vi "Facade.vi"(0 "Data In":T10 {"Duration (s)" format="%<%M:%S>T"}, 2 "Display State In":T8, 3 "Container State":T9) -> (6 "Data Out":T10 {"Duration (s)" format="%<%M:%S>T"}, 7 "Display State Out":T8, 8 "Action":T7)   [LabVIEW 2015, in "Song Browser.lvlib" / "Song Browser.xctl"]
uses:
  Song Browser.xctl
  Data.ctl
  controls/Queue Song Display.ctl
  file/MusicElement/Song/Song Duration.ctl
  controls/Dequeue Control.ctl
  <vilib>/_xctls/Container State.ctl
  State.ctl
  controls/Song Browser Display.ctl
  controls/Enqueue Control.ctl
  <vilib>/_xctls/Action.ctl
  controls/Ascending_Descending Order.ctl
  file/MusicElement/MusicElementLibrary/SongLibrary/Song Display Sort Option.ctl
  <vilib>/_xctls/XControlSupport.lvlib
  file/MusicElement/MusicElementLibrary/SongLibrary/SongLibrary.lvclass
  file/MusicElement/Song/Song.lvclass
panel:
  in  "Remove Filters":bool
  in  "Time Sort":bool
  out "Sort Time Indicator":T1
  out "Sort Album Indicator":T1
  in  "Album Sort":bool
  out "Sort Artist Indicator":T1
  in  "Artist Sort":bool
  in  "Song Sort":bool
  out "Sort Songs Indicator":T1
  out "Unfiltered Array":T2[](array[typedef]) {"Duration (s)" format="%<%M:%S>T"}
  in  "Array":T5[](array[typedef]) {"Duration (s)" format="%<%M:%S>T"}
  in  "Scrollbar":i32(c297)
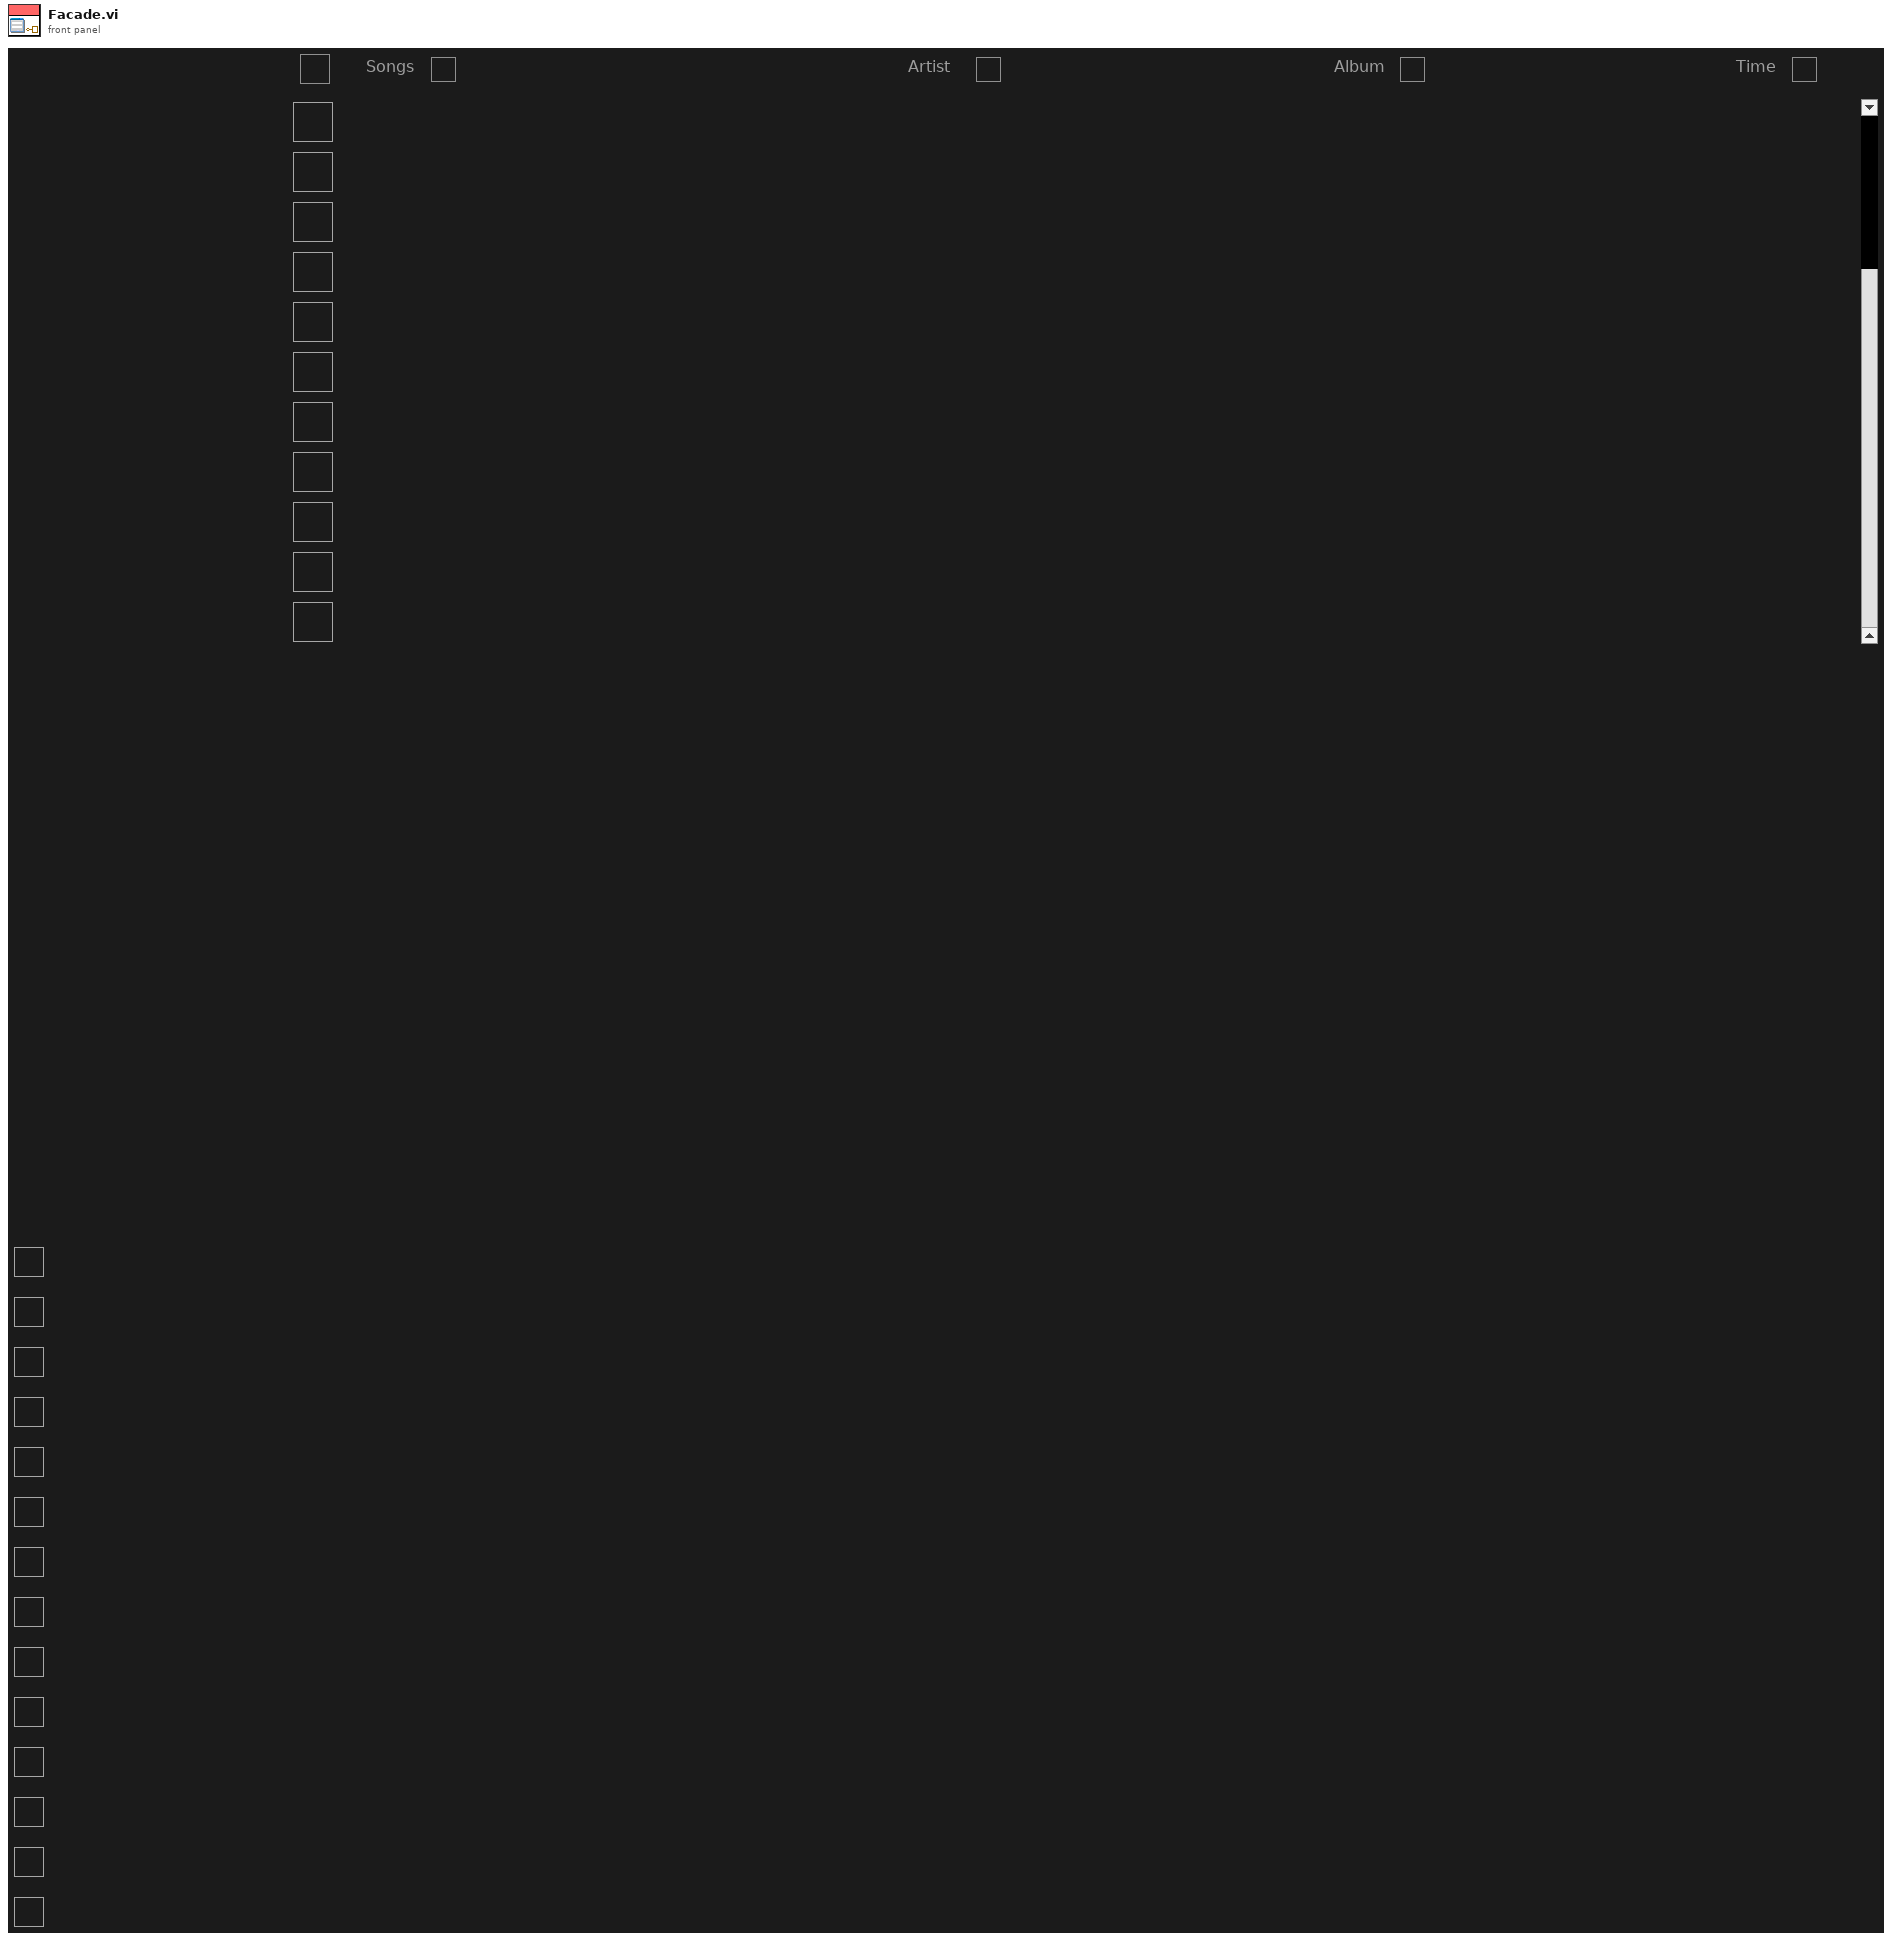
[diagram p1: front panel]
types:
  T1 = typedef "Ascending_Descending Order.ctl" = bool
  T2 = typedef "Queue Song Display.ctl" = cluster{"Song Name":string, "Artist":string, "Album":string, "Duration (s)":T3, "UID":string, "Dequeue":T4}
  T3 = typedef "Song.lvclass/Song Duration.ctl" = timestamp
  T4 = typedef "Dequeue Control.ctl" = bool
  T5 = typedef "Song Browser Display.ctl" = cluster{"Song Name":string, "Artist":string, "Album":string, "Duration (s)":T3, "UID":string, "Enqueue":T6}
  T6 = typedef "Enqueue Control.ctl" = bool
  T7 = typedef "XControlSupport.lvlib/Action.ctl" = cluster{"Data Changed?":bool, "State Changed?":bool, "Action Name":string}
  T8 = typedef "Song Browser.lvlib/Song Browser.xctl/State.ctl" = cluster{"Element Selected Event":refnum<user-event>}
  T9 = typedef "XControlSupport.lvlib/Container State.ctl" = cluster{"Indicator?":bool, "Run Mode?":bool, " Refnum":refnum<vi>}
  T10 = typedef "Song Browser.lvlib/Song Browser.xctl/Data.ctl" = T2[]
  T11 = cluster{"Song Name":bool, "Artist":bool, "Album":bool, "Duration (s)":bool, "UID":bool, "Enqueue":T6}
  T12 = typedef "SongLibrary.lvclass/Song Display Sort Option.ctl" = enum16{"Song", "Artist", "Album", "Time"}
  T13 = cluster{"Song Name":bool, "Artist":bool, "Album":bool, "Duration (s)":bool, "UID":bool, "Enqueue":T6}[]
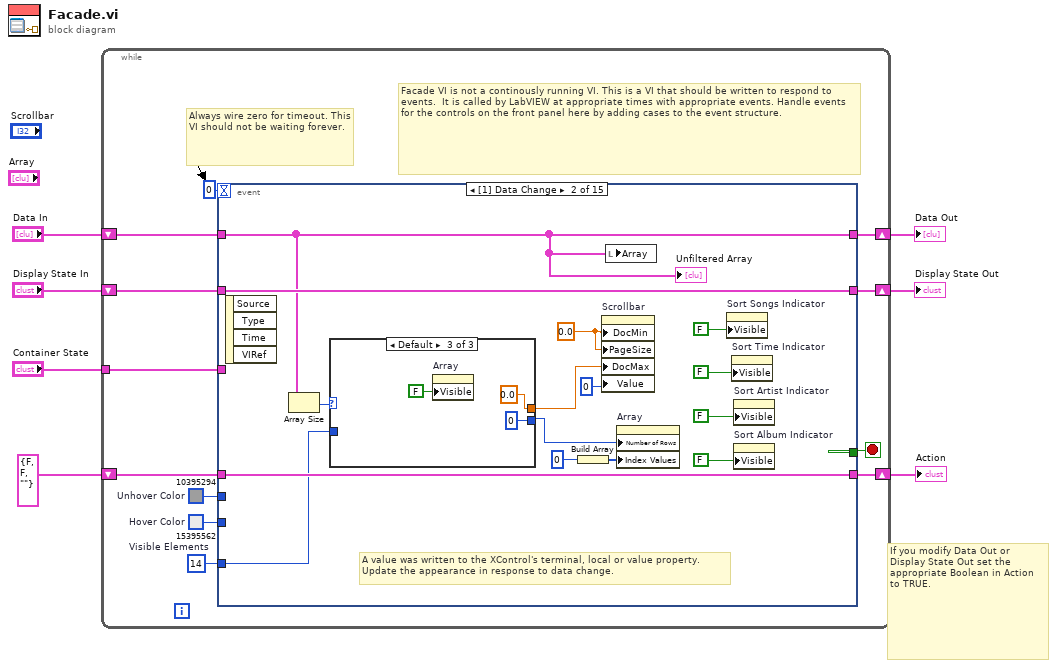
[diagram p0: block diagram]
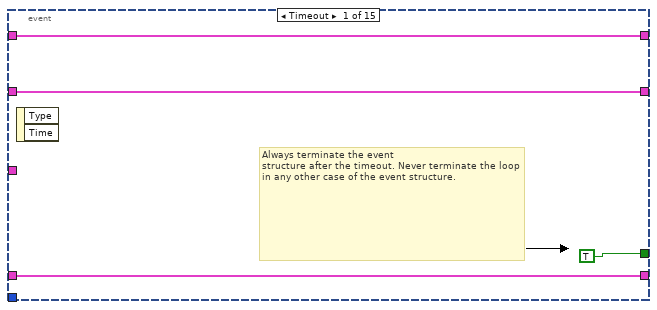
[diagram p2: hidden frame]
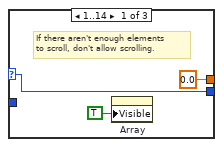
[diagram p3: hidden frame]
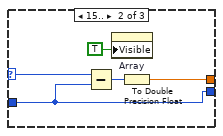
[diagram p4: hidden frame]
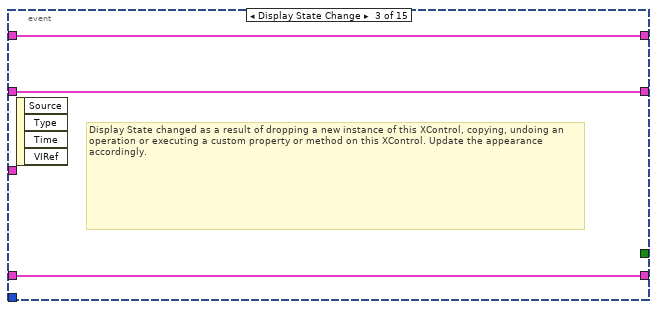
[diagram p5: hidden frame]
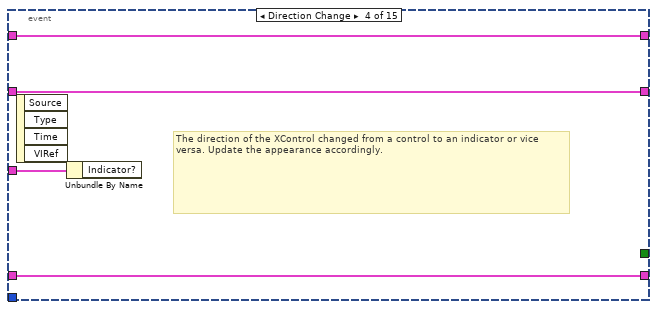
[diagram p6: hidden frame]
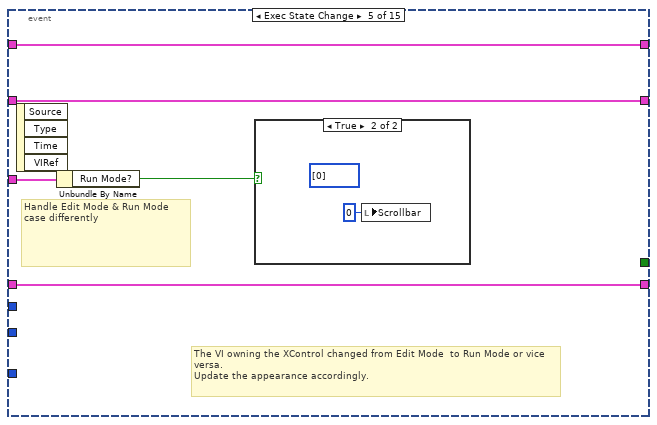
[diagram p7: hidden frame]
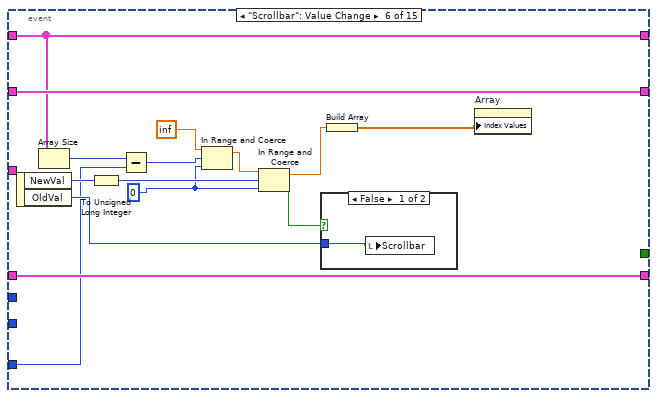
[diagram p9: hidden frame]
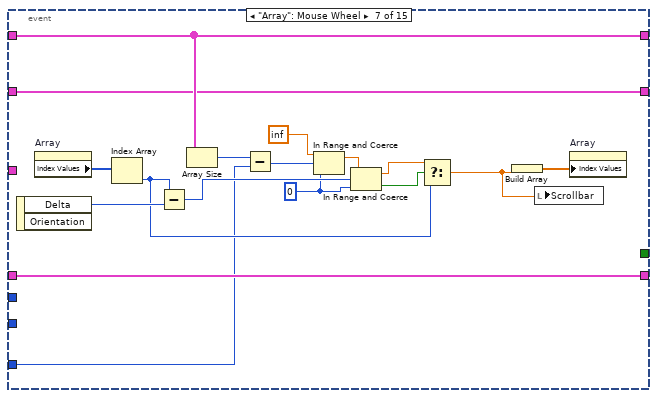
[diagram p11: hidden frame]
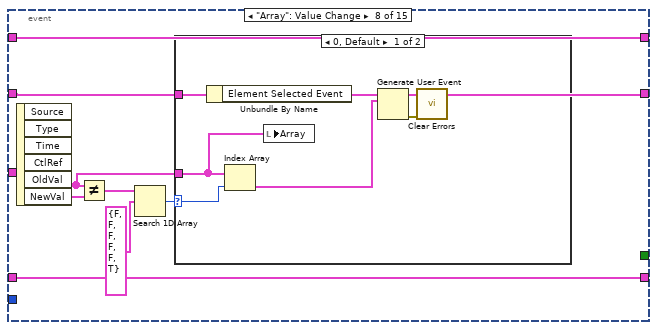
[diagram p12: hidden frame]
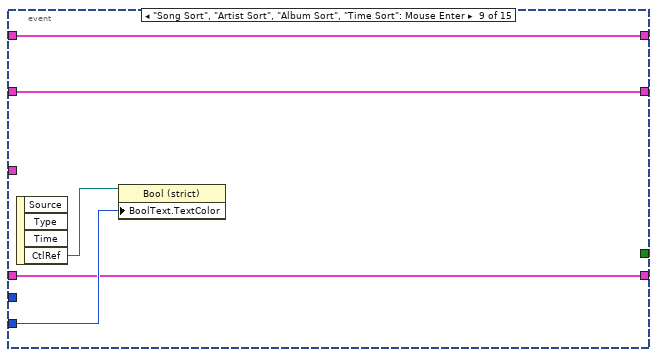
[diagram p14: hidden frame]
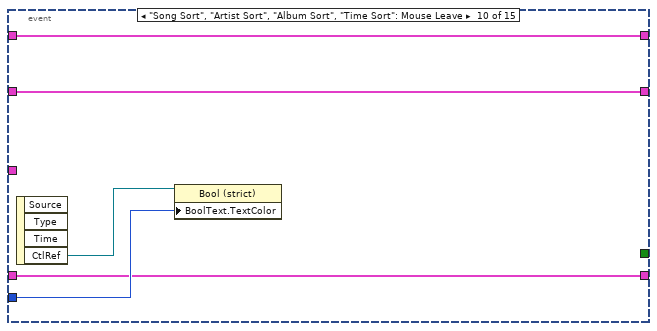
[diagram p15: hidden frame]
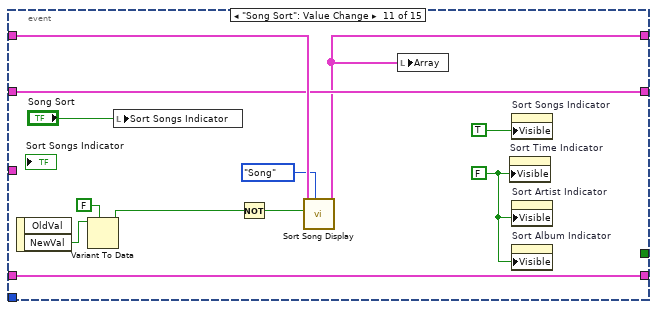
[diagram p16: hidden frame]
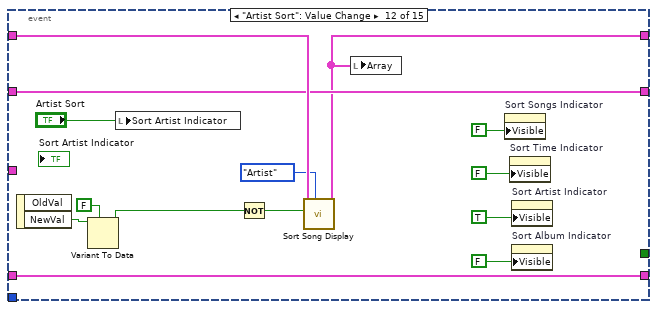
[diagram p17: hidden frame]
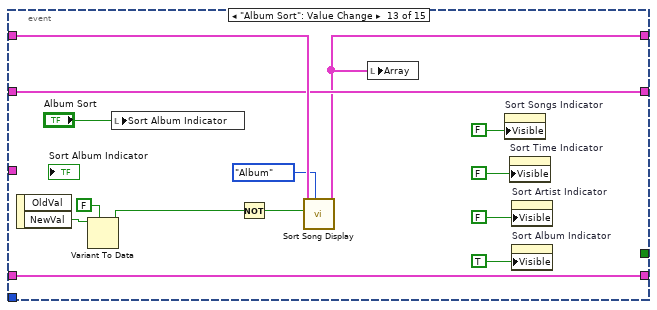
[diagram p18: hidden frame]
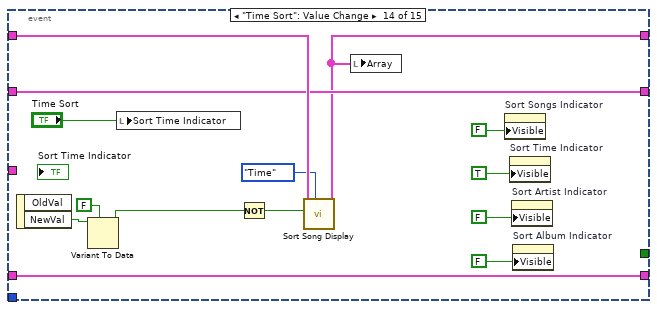
[diagram p19: hidden frame]
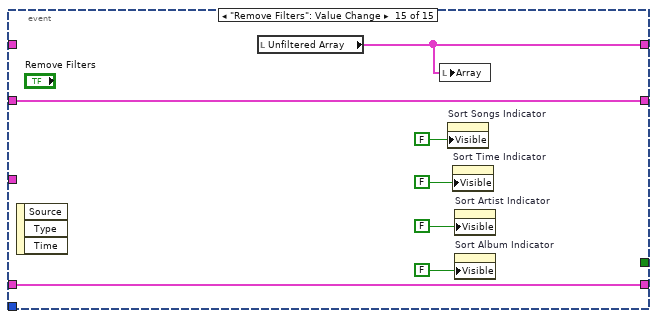
[diagram p20: hidden frame]
diagram:
  # "If you modify Data Out or\nDisplay State Out set the\nappropriate Boolean in Action\nto TRUE."
  n1 = while {
    shift-right: [w18] -> w3
    shift-left: "Display State In" -> [w19]
    tunnel: "Container State" -> [w15]
    shift-right: [w13] -> w2
    shift-left: "Data In" -> [w14]
    shift-right: [w11] -> w1
    shift-left: T7 {"Data Changed?"=FALSE, "State Changed?"=FALSE, "Action Name"=""} ("Action") -> [w12]
    stop <- w17 stop-if-true
    w8 = u32 15395562  # Hover Color
    w9 = u32 10395294  # Unhover Color
    w10 = 14  # Visible Elements
    # "Facade VI is not a continously running VI. This is a VI that should be written to respond to events.  It is called by LabVIEW at appropriate times with appropriate events. Handle events for the controls on the front panel here by adding cases to the event structure."
    # "Always wire zero for timeout. This\nVI should not be waiting forever."
    n2 = event shown="[1] Data Change" {
      selector: _ -> [_ _ _ _ _ _ _ _ _ _ _ _ _ _ _]
      dyn-events: _ -> [_ _ _ _ _ _ _ _ _ _ _ _ _ _ _]
      timeout: 0 -> [_ _ _ _ _ _ _ _ _ _ _ _ _ _ _]
      tunnel: w19 -> [w21 w28 w52 w55 w60 w75 w90 w99 w111 w116 w127 w142 w156 w170 w180]
      tunnel: [w21 w28 w52 w55 w60 w75 w90 w99 w111 w116 w127 w142 w156 w170 w180] -> w18
      tunnel: [TRUE _ _ _ _ _ _ _ _ _ _ _ _ _ _] -> w17
      tunnel: w15 -> [_ _ _ w56 w61 _ _ _ _ _ _ _ _ _ _]
      tunnel: w14 -> [w20 w27 w51 w54 w59 w73 w91 w103 w112 w115 w131 w145 w159 w173 _]
      tunnel: [w20 w27 w51 w54 w59 w73 w91 w103 w112 w115 w120 w132 w146 w160 w174] -> w13
      tunnel: [w22 w38 w50 w53 w58 w76 w92 w102 w110 w117 w126 w141 w155 w169 w179] -> w11
      tunnel: w12 -> [w22 w38 w50 w53 w58 w76 w92 w102 w110 w117 w126 w141 w155 w169 w179]
      tunnel: w10 -> [_ w36 _ _ _ w68 w86 _ _ _ _ _ _ _ _]
      tunnel: w9 -> [_ _ _ _ _ _ _ _ _ w118 _ _ _ _ _]
      tunnel: w8 -> [_ _ _ _ _ _ _ _ w113 _ _ _ _ _ _]
      event Timeout {
        # "Always terminate the event\nstructure after the timeout. Never terminate the loop in any other case of the event structure."
        n3 = event-data() -> ()  [unwired: 1 in, 2 out]
      }
      event Data Change {
        w31 = 0.0 ("Doc Min")
        # "A value was written to the XControl's terminal, local or value property.\nUpdate the appearance in response to data change."
        n4 = event-data() -> ()  [unwired: 1 in, 4 out]
        n5 = Array Size(array=w27) -> (size(s)=w37:i32)
        n6 = case shown="Default" w37 {
          selector: w37 -> [w41 w45 _]
          tunnel: [w41 w43 0 ("y")] -> w29
          tunnel: [0.0 ("Doc Min") w46 0.0 ("Doc Max")] -> w30
          tunnel: w36 -> [_ w43 _]
          frame 1..14 {
            # "If there aren't enough elements\nto scroll, don't allow scrolling."
            n7 = property on="Array" class="Arr"("Visible"=TRUE) -> ()  [unwired: 2 in, 2 out]
          }
          frame 15.. {
            n8 = Subtract(x=w45, y=w43) -> (x-y=w44:i32)
            n9 = property on="Array" class="Arr"("Visible"=TRUE) -> ()  [unwired: 2 in, 2 out]
            n10 = To Double Precision Float(number=w44) -> (double precision float=w46:dbl)
          }
          frame Default {
            n11 = property on="Array" class="Arr"("Visible"=FALSE) -> ()  [unwired: 2 in, 2 out]
          }
        }
        n12 = Build Array(0 ("y")) -> (w25:i32[])
        n13 = property on="Scrollbar" class="Scroll (strict)"("DocMin"=w31, "PageSize"=w31, "DocMax"=w30, "Value"=0 ("y")) -> ()  [unwired: 2 in, 2 out]
        n14 = local write "Array"(w27) -> ()
        n15 = property on="Array" class="Arr"("Number of Rows"=w29, "Index Values"=w25) -> ()  [unwired: 2 in, 2 out]
        n16 = property on="Sort Songs Indicator" class="Bool (strict)"("Visible"=FALSE) -> ()  [unwired: 2 in, 2 out]
        n17 = property on="Sort Time Indicator" class="Bool (strict)"("Visible"=FALSE) -> ()  [unwired: 2 in, 2 out]
        n18 = property on="Sort Artist Indicator" class="Bool (strict)"("Visible"=FALSE) -> ()  [unwired: 2 in, 2 out]
        n19 = property on="Sort Album Indicator" class="Bool (strict)"("Visible"=FALSE) -> ()  [unwired: 2 in, 2 out]
        "Unfiltered Array" <- w27
      }
      event Display State Change {
        # "Display State changed as a result of dropping a new instance of this XControl, copying, undoing an operation or executing a custom property or method on this XControl. Update the appearance accordingly."
        n20 = event-data() -> ()  [unwired: 1 in, 4 out]
      }
      event Direction Change {
        # "The direction of the XControl changed from a control to an indicator or vice versa. Update the appearance accordingly."
        n21 = event-data() -> ()  [unwired: 1 in, 4 out]
        n22 = Unbundle By Name(w56) -> ()  [unwired: 1 out]
      }
      event Exec State Change {
        # "The VI owning the XControl changed from Edit Mode  to Run Mode or vice versa.\nUpdate the appearance accordingly."
        # "Handle Edit Mode & Run Mode\ncase differently"
        n23 = event-data() -> ()  [unwired: 1 in, 4 out]
        n24 = Unbundle By Name(w61) -> ("Run Mode?"=w57:bool)
        n25 = case shown="True" w57 {
          frame False {
          }
          frame True {
            (unwired) u32[] [0] ("Index Values")
            n26 = local write "Scrollbar"(0 ("Scrollbar")) -> ()
          }
        }
      }
      event "Scrollbar": Value Change {
        w64 = u32 0 ("upper limit")
        n27 = event-data() -> ("NewVal"=w77:i32, "OldVal"=w69:i32)  [unwired: 1 in]
        n28 = Array Size(array=w73) -> (size(s)=w72:i32)
        n29 = To Unsigned Long Integer(number=w77) -> (unsigned 32bit integer=w74:u32)
        n30 = Subtract(x=w72, y=w68) -> (x-y=w65:i32)
        n31 = In Range and Coerce(upper limit=inf, x=w65, lower limit=w64) -> (coerced(x)=w63:dbl)  [unwired: 1 out]
        n32 = In Range and Coerce(upper limit=w63, x=w74, lower limit=w64) -> (coerced(x)=w71:dbl, In Range?=w70:bool)
        n33 = case shown="False" w70 {
          tunnel: w69 -> [w78 _]
          frame False {
            n34 = local write "Scrollbar"(w78) -> ()
          }
          frame True {
          }
        }
        n35 = Build Array(w71) -> (w67:dbl[])
        n36 = property on="Array" class="Arr"("Index Values"=w67) -> ()  [unwired: 2 in, 2 out]
      }
      event "Array": Mouse Wheel {
        w79 = u32 0 ("upper limit")
        n37 = event-data() -> ("Delta"=w95:i32)  [unwired: 1 in, 1 out]
        n38 = property on="Array" class="Arr"() -> ("Index Values"=w83:u32[])  [unwired: 2 in, 2 out]
        n39 = Index Array(array=w83) -> (element=w87:u32)  [unwired: 1 in]
        n40 = Subtract(x=w87, y=w95) -> (x-y=w93:u32)
        n41 = Array Size(array=w91) -> (size(s)=w94:i32)
        n42 = Subtract(x=w94, y=w86) -> (x-y=w80:i32)
        n43 = In Range and Coerce(upper limit=inf, x=w80, lower limit=w79) -> (coerced(x)=w81:dbl)  [unwired: 1 out]
        n44 = In Range and Coerce(upper limit=w81, x=w93, lower limit=w79) -> (coerced(x)=w88:dbl, In Range?=w89:bool)
        n45 = Select(t=w88, s=w89, f=w87) -> (s? t:f=w85:dbl)
        n46 = Build Array(w85) -> (w84:dbl[])
        n47 = local write "Scrollbar"(w85) -> ()
        n48 = property on="Array" class="Arr"("Index Values"=w84) -> ()  [unwired: 2 in, 2 out]
      }
      event "Array": Value Change {
        n49 = event-data() -> ("OldVal"=w96:T5[], "NewVal"=w97:T5[])  [unwired: 1 in, 4 out]
        n50 = Not Equal?(x=w96, y=w97) -> (x != y?=w101:T13)
        n51 = Search 1D Array(1D array=w101, element=T11 {"Song Name"=FALSE, "Artist"=FALSE, "Album"=FALSE, "Duration (s)"=FALSE, "UID"=FALSE, "Enqueue"=TRUE}) -> (index of element=w100:i32)  [unwired: 1 in]
        n52 = case shown="0, Default" w100 {
          selector: w100 -> [w107 _]
          tunnel: w99 -> [w109 _]
          tunnel: w96 -> [w104 _]
          frame 0, Default {
            n53 = Unbundle By Name(w109) -> ("Element Selected Event"=w106:refnum<user-event>)
            n54 = Index Array(array=w104, index=w107) -> (element=w105:T5)
            n55 = local write "Array"(w104) -> ()
            n56 = Generate User Event(user event=w106, event data cluster=w105) -> (error out=w108:errorcluster)  [unwired: 2 in, 1 out]
            n57 = call <vilib>:"Clear Errors.vi"("error in (no error)"=w108) -> ()  [unwired: 5 in, 2 out]
          }
          frame ..-1 {
          }
        }
      }
      event "Song Sort", "Artist Sort", "Album Sort", "Time Sort": Mouse Enter {
        n58 = event-data() -> ("CtlRef"=w114:refnum<vi>)  [unwired: 1 in, 3 out]
        n59 = property class="Bool (strict)"(reference=w114, "BoolText.TextColor"=w113) -> ()  [unwired: 1 in, 2 out]
      }
      event "Song Sort", "Artist Sort", "Album Sort", "Time Sort": Mouse Leave {
        n60 = event-data() -> ("CtlRef"=w119:refnum<vi>)  [unwired: 1 in, 3 out]
        n61 = property class="Bool (strict)"(reference=w119, "BoolText.TextColor"=w118) -> ()  [unwired: 1 in, 2 out]
      }
      event "Song Sort": Value Change {
        w124 = FALSE ("Visible")
        n62 = event-data() -> ("NewVal"=w121:bool)  [unwired: 1 in, 1 out]
        n63 = Variant To Data(type=T1 FALSE ("Sort Songs Indicator"), Variant=w121) -> (data=w122:T1)  [unwired: 1 in, 1 out]
        n64 = local write "Sort Songs Indicator"("Song Sort") -> ()
        n65 = Not(x=w122) -> (.not. x?=w123:T1)
        n66 = call "Sort Song Display.vi"("Options"=Song_Display_Sort_Option."Song", "Reverse?"=w123, "Songs"=w131) -> ("Sorted Songs"=w120:T2[])  [unwired: 7 in, 1 out]
        n67 = local write "Array"(w120) -> ()
        n68 = property on="Sort Time Indicator" class="Bool (strict)"("Visible"=w124) -> ()  [unwired: 2 in, 2 out]
        n69 = property on="Sort Songs Indicator" class="Bool (strict)"("Visible"=TRUE) -> ()  [unwired: 2 in, 2 out]
        n70 = property on="Sort Artist Indicator" class="Bool (strict)"("Visible"=w124) -> ()  [unwired: 2 in, 2 out]
        n71 = property on="Sort Album Indicator" class="Bool (strict)"("Visible"=w124) -> ()  [unwired: 2 in, 2 out]
      }
      event "Artist Sort": Value Change {
        n72 = event-data() -> ("NewVal"=w133:bool)  [unwired: 1 in, 1 out]
        n73 = Variant To Data(type=T1 FALSE ("Sort Songs Indicator"), Variant=w133) -> (data=w138:T1)  [unwired: 1 in, 1 out]
        n74 = local write "Sort Artist Indicator"("Artist Sort") -> ()
        n75 = Not(x=w138) -> (.not. x?=w139:T1)
        n76 = call "Sort Song Display.vi"("Options"=Song_Display_Sort_Option."Artist", "Reverse?"=w139, "Songs"=w145) -> ("Sorted Songs"=w132:T2[])  [unwired: 7 in, 1 out]
        n77 = local write "Array"(w132) -> ()
        n78 = property on="Sort Songs Indicator" class="Bool (strict)"("Visible"=FALSE) -> ()  [unwired: 2 in, 2 out]
        n79 = property on="Sort Time Indicator" class="Bool (strict)"("Visible"=FALSE) -> ()  [unwired: 2 in, 2 out]
        n80 = property on="Sort Artist Indicator" class="Bool (strict)"("Visible"=TRUE) -> ()  [unwired: 2 in, 2 out]
        n81 = property on="Sort Album Indicator" class="Bool (strict)"("Visible"=FALSE) -> ()  [unwired: 2 in, 2 out]
      }
      event "Album Sort": Value Change {
        n82 = event-data() -> ("NewVal"=w149:bool)  [unwired: 1 in, 1 out]
        n83 = Variant To Data(type=T1 FALSE ("Sort Songs Indicator"), Variant=w149) -> (data=w152:T1)  [unwired: 1 in, 1 out]
        n84 = local write "Sort Album Indicator"("Album Sort") -> ()
        n85 = Not(x=w152) -> (.not. x?=w153:T1)
        n86 = call "Sort Song Display.vi"("Options"=Song_Display_Sort_Option."Album", "Reverse?"=w153, "Songs"=w159) -> ("Sorted Songs"=w146:T2[])  [unwired: 7 in, 1 out]
        n87 = local write "Array"(w146) -> ()
        n88 = property on="Sort Songs Indicator" class="Bool (strict)"("Visible"=FALSE) -> ()  [unwired: 2 in, 2 out]
        n89 = property on="Sort Time Indicator" class="Bool (strict)"("Visible"=FALSE) -> ()  [unwired: 2 in, 2 out]
        n90 = property on="Sort Artist Indicator" class="Bool (strict)"("Visible"=FALSE) -> ()  [unwired: 2 in, 2 out]
        n91 = property on="Sort Album Indicator" class="Bool (strict)"("Visible"=TRUE) -> ()  [unwired: 2 in, 2 out]
      }
      event "Time Sort": Value Change {
        n92 = event-data() -> ("NewVal"=w164:bool)  [unwired: 1 in, 1 out]
        n93 = Variant To Data(type=T1 FALSE ("Sort Songs Indicator"), Variant=w164) -> (data=w166:T1)  [unwired: 1 in, 1 out]
        n94 = local write "Sort Time Indicator"("Time Sort") -> ()
        n95 = Not(x=w166) -> (.not. x?=w167:T1)
        n96 = call "Sort Song Display.vi"("Options"=Song_Display_Sort_Option."Time", "Reverse?"=w167, "Songs"=w173) -> ("Sorted Songs"=w160:T2[])  [unwired: 7 in, 1 out]
        n97 = local write "Array"(w160) -> ()
        n98 = property on="Sort Songs Indicator" class="Bool (strict)"("Visible"=FALSE) -> ()  [unwired: 2 in, 2 out]
        n99 = property on="Sort Time Indicator" class="Bool (strict)"("Visible"=TRUE) -> ()  [unwired: 2 in, 2 out]
        n100 = property on="Sort Artist Indicator" class="Bool (strict)"("Visible"=FALSE) -> ()  [unwired: 2 in, 2 out]
        n101 = property on="Sort Album Indicator" class="Bool (strict)"("Visible"=FALSE) -> ()  [unwired: 2 in, 2 out]
      }
      event "Remove Filters": Value Change {
        n102 = event-data() -> ()  [unwired: 1 in, 3 out]
        n103 = local read "Unfiltered Array"() -> (w174:T2[])
        n104 = local write "Array"(w174) -> ()
        n105 = property on="Sort Songs Indicator" class="Bool (strict)"("Visible"=FALSE) -> ()  [unwired: 2 in, 2 out]
        n106 = property on="Sort Time Indicator" class="Bool (strict)"("Visible"=FALSE) -> ()  [unwired: 2 in, 2 out]
        n107 = property on="Sort Artist Indicator" class="Bool (strict)"("Visible"=FALSE) -> ()  [unwired: 2 in, 2 out]
        n108 = property on="Sort Album Indicator" class="Bool (strict)"("Visible"=FALSE) -> ()  [unwired: 2 in, 2 out]
      }
    }
  }
  "Display State Out" <- w3
  "Data Out" <- w2
  "Action" <- w1
